vi "IntakeLower.vi"(7 "Description":string, 8 "Command Info In":T1) -> (0 "Command Info Out":T1)   [LabVIEW 2017]
doc: "This template is useful for immediate subsystem actions that do not need deadband filtering\n\nBe sure to right-click and select New from Template and save with a new command name."
uses:
  <vilib>/Rock Robotics/WPI/Framework/Command Status Info.ctl
  <vilib>/Rock Robotics/WPI/Framework/Completion Status.ctl
  <vilib>/Rock Robotics/WPI/Framework/Completion Notifier.ctl
  Implementation/Intake Setpoints.ctl
  Implementation/Intake Operations.ctl
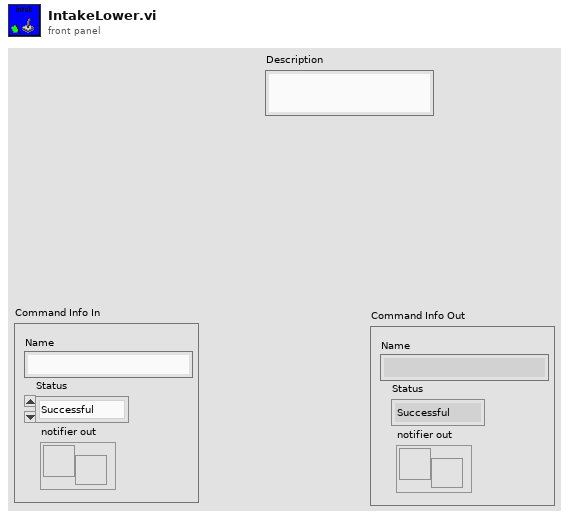
[diagram p1: front panel]
types:
  T1 = typedef "Command Status Info.ctl" = cluster{"Name":string, "Status":T2, "notifier out":T3}
  T2 = typedef "Completion Status.ctl" = enum16{"Successful", "Aborted", "Incomplete"}
  T3 = typedef "Completion Notifier.ctl" = refnum<notifier>
  T4 = typedef "Intake Operations.ctl" = enum16{"idle", "setSetpoint", "feed", "spit"}
  T5 = typedef "Intake Setpoints.ctl" = cluster{"Operation":T4, "Degree Setpoint":dbl}
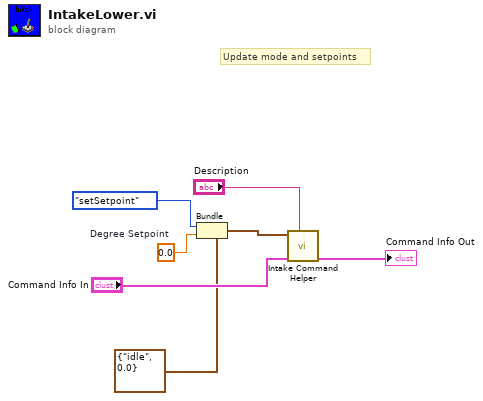
[diagram p0: block diagram]
diagram:
  w2 = 0.0  # Degree Setpoint
  # "Update mode and setpoints"
  n1 = Bundle(cluster=T5 {"Operation"=enum."idle", "Degree Setpoint"=0.0} ("SubSystem Data"), "Operation"=Intake_Operations."setSetpoint", "Degree Setpoint"=w2) -> (w3:T5)
  n2 = call "Intake Command Helper.vi"("Description"="Description", "Command Info In"="Command Info In", "SubSystem Data"=w3) -> ("Command Info Out"=→"Command Info Out":T1)  [unwired: 6 in, 2 out]
